vi "Actor Core.vi"(8 "error in":errorcluster, 11 "Main in":refnum<class "Main.lvclass">) -> (0 "error out":errorcluster, 3 "Actor out":refnum<class "Actor.lvclass">)   [LabVIEW 2025, in "Main.lvlib" / "Main.lvclass"]
doc: "<p>(<strong>Filename</strong>: <span class=\"dnl\">Actor Framework.lvlib:Actor.lvclass:Actor Core.vi</span>)</p>\n<p>Receives messages to the actor, reacts to them, and initiates any error handling that may shut the actor down.</p>\n<p>Descendant classes may override this VI to append parallel tasks for the actor to complete while it handles messages. Overrides use the <a href=\"nihelplauncher://docs/csh?context=lvcore_glang_udclass\">Call Parent Class Method</a> node.</p>"
uses:
  Main.lvclass
  C:/Program Files/National Instruments/LabVIEW 2025/vi.lib/ActorFramework/Actor/Actor.lvclass
  C:/Program Files/National Instruments/LabVIEW 2025/vi.lib/MGI/Panel Manager/Panel Actor/Panel Actor/Panel Actor.lvclass
  <vilib>/ActorFramework/Actor/Actor.lvclass
  File Worker/File Worker/File Worker.lvclass
  Main.lvclass/Main.ctl
  <vilib>/ActorFramework/Message Enqueuer/Message Enqueuer.lvclass/Message Enqueuer.ctl
  File Worker/File Worker Messages/Start Write Action Msg/Start Write Action Msg.lvclass/Start Write Action Msg.ctl
  File Worker/File Worker Messages/Start Read Action Msg/Start Read Action Msg.lvclass/Start Read Action Msg.ctl
  08b86284-690f-4d6a-a57b-caf26b63b25f.vi
  <vilib>/ActorFramework/Message Enqueuer/Enqueue.vi
  <vilib>/ActorFramework/Stop Msg/Stop Msg.lvclass
  C:/Program Files/National Instruments/LabVIEW 2025/vi.lib/ActorFramework/Message/Message.lvclass
  Main Messages/Reset Write Statistics Msg/Reset Write Statistics Msg.lvclass
  File Worker/File Worker Messages/Start Write Action Msg/Start Write Action Msg.lvclass
  Main Messages/Reset Read Statistics Msg/Reset Read Statistics Msg.lvclass
  File Worker/File Worker Messages/Start Read Action Msg/Start Read Action Msg.lvclass
  <vilib>/ActorFramework/Message Priority Queue/Priority Enqueue.vi
  <vilib>/Platform/browser.llb/Open URL in Default Browser (string).vi
  <vilib>/MGI/Panel Manager/Panel Actor/Panel Actor/Panel Actor.lvclass
panel:
  in  "Visit RADX":bool
  in  "Visit G2CPU":bool
  in  "Stop Action":bool
  in  "Read":bool
  in  "Write":bool
  in  "Block Size":u16(ring)
  in  "Threads":i32=4 min=1 step=1
  in  "File Size":u16(ring)
  in  "Available Disks":u16(ring)
  out "Write Average":dbl format="%#_2g GB/s"
  out "Write Min":dbl format="%#_2g GB/s"
  out "Write Max":dbl format="%#_2g GB/s"
  out "Write Plot":waveform(dbl)(graph)
  out "Read Average":dbl format="%#_2g GB/s"
  out "Read Min":dbl format="%#_2g GB/s"
  out "Read Max":dbl format="%#_2g GB/s"
  out "Read Plot":waveform(dbl)(graph)
  # "GPU acceleration in LabVIEW?"
  # "Sponsored by:"
  # "COTS, High Performance PXIe Data Storage, GPU and GbE"
  # "Copyright 2025 G2CPU, Ltd. \nAll Rights Reserved."
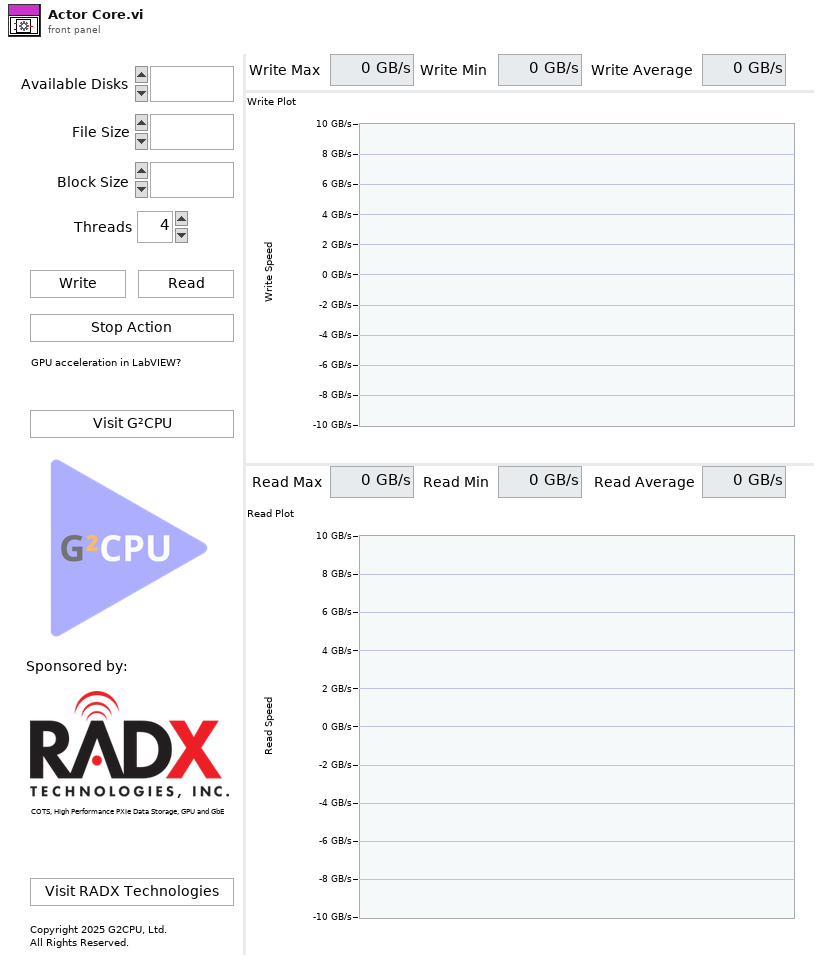
[diagram p1: front panel]
types:
  T1 = enum32{"Invalid", "Standard", "Closed", "Hidden", "Minimized", "Maximized"}
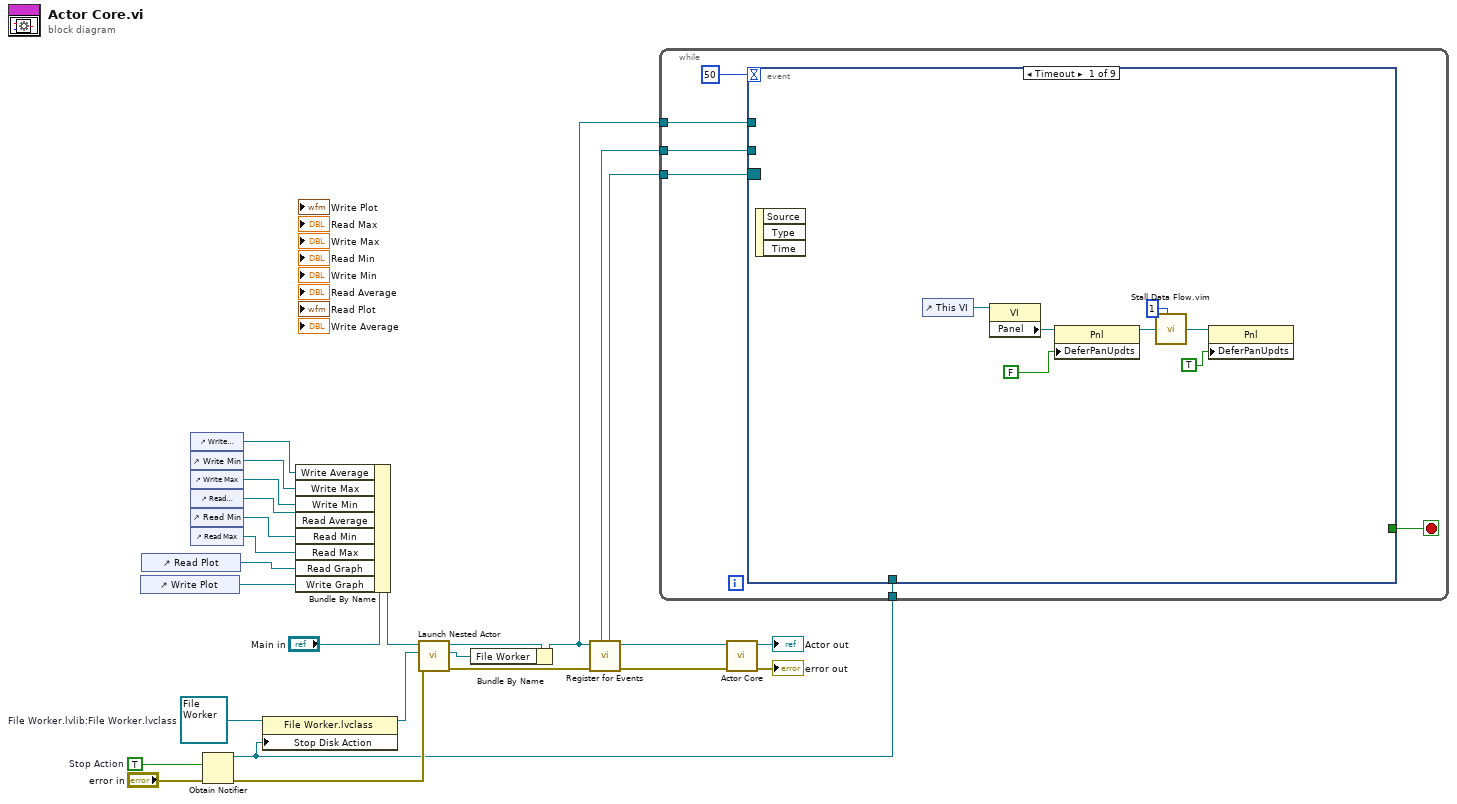
[diagram p0: block diagram]
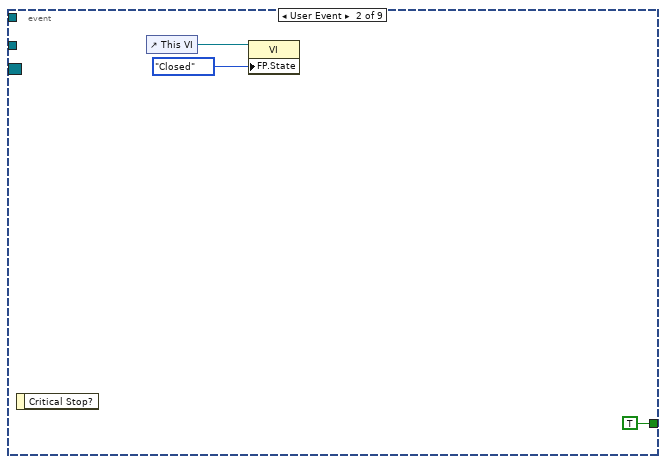
[diagram p2: hidden frame]
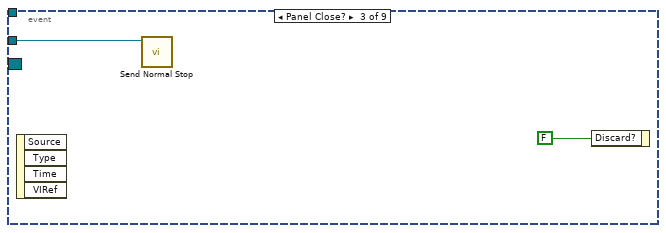
[diagram p3: hidden frame]
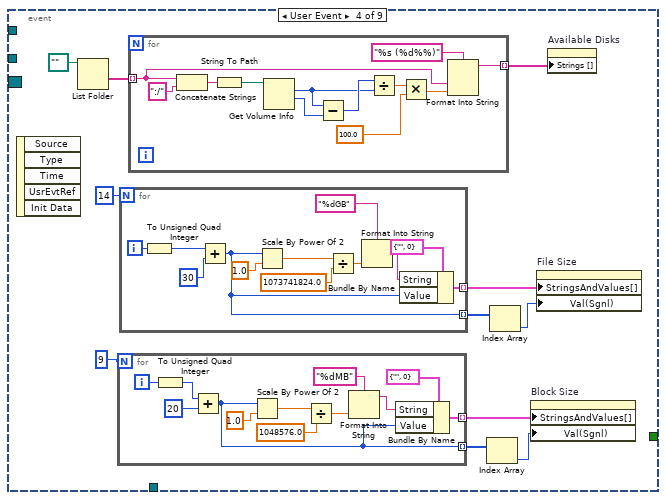
[diagram p4: hidden frame]
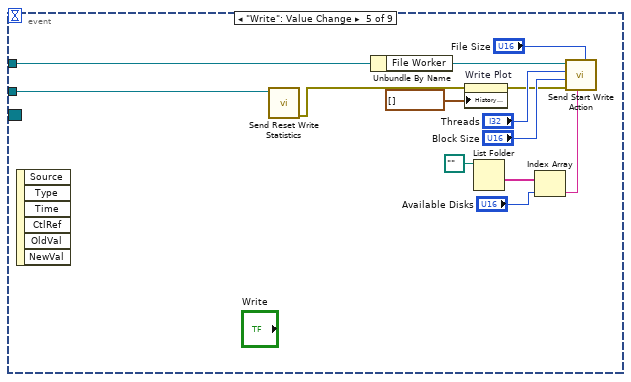
[diagram p5: hidden frame]
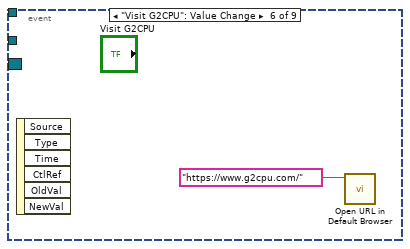
[diagram p6: hidden frame]
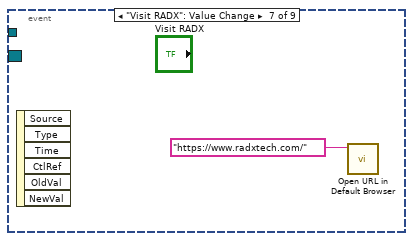
[diagram p7: hidden frame]
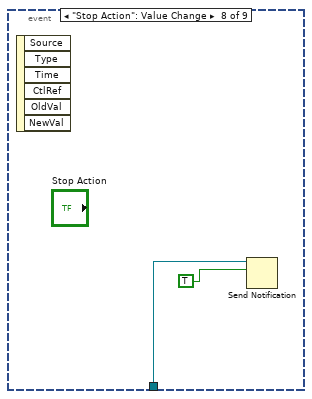
[diagram p8: hidden frame]
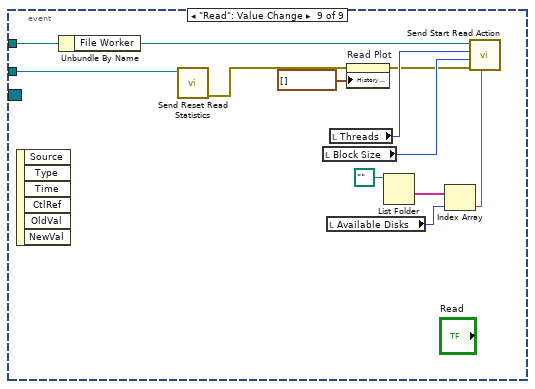
[diagram p9: hidden frame]
diagram:
  w11 = TRUE  # Stop Action
  w17 = refnum<class "File Worker.lvclass"> refnum  # File Worker.lvlib:File Worker.lvclass
  n1 = control-ref of="Write Plot"() -> (w13:refnum<vi>)
  n2 = control-ref of="Read Plot"() -> (w12:refnum<vi>)
  n3 = control-ref of="Write Average"() -> (w6:refnum<vi>)
  n4 = control-ref of="Write Min"() -> (w5:refnum<vi>)
  n5 = control-ref of="Write Max"() -> (w4:refnum<vi>)
  n6 = control-ref of="Read Average"() -> (w3:refnum<vi>)
  n7 = control-ref of="Read Min"() -> (w2:refnum<vi>)
  n8 = control-ref of="Read Max"() -> (w1:refnum<vi>)
  n9 = Obtain Notifier(notification data type=w11, error in (no error)="error in") -> (notifier out=w7:refnum<notifier>, error out=w9:errorcluster)  [unwired: 2 in, 1 out]
  n10 = property class="File Worker.lvclass"(reference=w17, "Stop Disk Action"=w7) -> (reference out=w8:refnum<class "File Worker.lvclass">)  [unwired: 1 in, 1 out]
  n11 = Bundle By Name(cluster="Main in", "Write Average"=w6, "Write Max"=w5, "Write Min"=w4, "Read Average"=w3, "Read Min"=w2, "Read Max"=w1, "Read Graph"=w12, "Write Graph"=w13) -> (w14:refnum<class "Main.lvclass">)
  n12 = call <vilib>:"Launch Nested Actor.vi"("error in (no error)"=w9, "Nested Actor"=w8, "Caller Actor in"=w14) -> ("error out"=w20:errorcluster, "Nested Actor's Enqueuer"=w16:refnum<class "Message Enqueuer.lvclass">, "Caller Actor out"=w18:refnum<class "Main.lvclass">)  [unwired: 6 in]
  n13 = Bundle By Name(cluster=w18, "File Worker"=w16) -> (w15:refnum<class "Main.lvclass">)
  n14 = call <vilib>:"Register for Events.vi"("Error In"=w20, "Panel Actor in"=w15) -> ("Error Out"=w23:errorcluster, "Panel Actor out"=w24:refnum<class "Main.lvclass">, "Pnl Actor"=w22:refnum<event-registration>, "Self Enqueuer"=w21:refnum<class "Message Enqueuer.lvclass">)  [unwired: 6 in]
  n15 = while {
    tunnel: w22 -> [w32]
    tunnel: w21 -> [w30]
    tunnel: w15 -> [w29]
    tunnel: w7 -> [w28]
    stop <- w31 stop-if-true
    n16 = event shown="[0] Timeout" {
      selector: w32 -> [_ _ _ _ _ _ _ _ _]
      dyn-events: _ -> [_ _ _ _ _ _ _ _ _]
      timeout: 50 -> [_ _ _ _ _ _ _ _ _]
      tunnel: [_ TRUE _ _ _ _ _ _ _] -> w31
      tunnel: w30 -> [_ _ w43 _ w93 _ _ _ w109]
      tunnel: w29 -> [_ _ _ _ w104 _ _ _ w120]
      tunnel: w28 -> [_ _ _ _ _ _ _ w108 _]
      event Timeout {
        n17 = event-data() -> ()  [unwired: 1 in, 3 out]
        n18 = control-ref of="This VI"() -> (w38:refnum<vi>)
        n19 = property class="VI"(reference=w38) -> ("Panel"=w39:refnum<vi>)  [unwired: 1 in, 2 out]
        n20 = property class="Pnl"(reference=w39, "DeferPanUpdts"=FALSE ("Defer Panel Updates")) -> (reference out=w36:refnum<vi>)  [unwired: 1 in, 1 out]
        n21 = call "Stall Data Flow.vim"("value in"=w36, "milliseconds to wait"=u32 1) -> ("value out"=w34:refnum<vi>)  [unwired: 1 out]
        n22 = property class="Pnl"(reference=w34, "DeferPanUpdts"=TRUE ("Defer Panel Updates")) -> ()  [unwired: 1 in, 2 out]
      }
      event User Event {
        n23 = event-data() -> ()  [unwired: 1 in, 1 out]
        n24 = control-ref of="This VI"() -> (w41:refnum<vi>)
        n25 = property class="VI"(reference=w41, "FP.State"=T1."Closed" ("Front Panel Window:State")) -> ()  [unwired: 1 in, 2 out]
      }
      event Panel Close? {
        n26 = event-data() -> ()  [unwired: 1 in, 4 out]
        n27 = call <vilib>:"Send Normal Stop.vi"("Message Enqueuer"=w43) -> ()  [unwired: 10 in, 1 out]
        n28 = event-data("Discard?"=FALSE) -> ()  [unwired: 1 in, 1 out]
      }
      event User Event {
        n29 = event-data() -> ()  [unwired: 1 in, 5 out]
        n30 = List Folder(path=path "") -> (folder names=w54:string[])  [unwired: 3 in, 3 out]
        n31 = for {
          N: 9 -> [_]
          tunnel: [w58] -> w47 mode=indexing
          tunnel: [w56] -> w45 mode=indexing
          i -> [w62]
          n32 = To Unsigned Quad Integer(1:w62) -> (0:w57:u64)
          n33 = Add(x=w57, y=u64 20) -> (x+y=w56:u64)
          n34 = Scale By Power Of 2(n=w56, x=1.0 ("y")) -> (x*2^n=w67:dbl)
          n35 = Divide(x=w67, y=1048576.0 ("x")) -> (x/y=w61:dbl)
          n36 = Format Into String(format string="%dMB", w61) -> (resulting string=w59:string)  [unwired: 2 in, 1 out]
          n37 = Bundle By Name(cluster=cluster{"String":string, "Value":u16} {"String"="", "Value"=0} ("element"), "String"=w59, "Value"=w56) -> (w58:cluster{"String":string, "Value":u16})
        }
        n38 = for {
          N: 14 -> [_]
          tunnel: [w72] -> w51 mode=indexing
          tunnel: [w69] -> w50 mode=indexing
          i -> [w78]
          n39 = To Unsigned Quad Integer(1:w78) -> (0:w68:u64)
          n40 = Add(x=w68, y=u64 30) -> (x+y=w69:u64)
          n41 = Scale By Power Of 2(n=w69, x=1.0 ("y")) -> (x*2^n=w73:dbl)
          n42 = Divide(x=w73, y=1073741824.0 ("x")) -> (x/y=w71:dbl)
          n43 = Format Into String(format string="%dGB", w71) -> (resulting string=w74:string)  [unwired: 2 in, 1 out]
          n44 = Bundle By Name(cluster=cluster{"String":string, "Value":u16} {"String"="", "Value"=0} ("element"), "String"=w74, "Value"=w69) -> (w72:cluster{"String":string, "Value":u16})
        }
        n45 = for {
          tunnel: w54 -> [w82] mode=indexing
          tunnel: [w80] -> w53 mode=indexing
          n46 = Concatenate Strings(w82, ":/" ("string")) -> (w90:string)
          n47 = String To Path(string=w90) -> (path=w91:path)
          n48 = Get Volume Info(11:w91) -> (1:w88:i64, 2:w86:i64)  [unwired: 1 in, 4 out]
          n49 = Subtract(x=w86, y=w88) -> (x-y=w87:i64)
          n50 = Divide(x=w87, y=w86) -> (x/y=w85:dbl)
          n51 = Multiply(x=w85, y=100.0) -> (x*y=w81:dbl)
          n52 = Format Into String(format string="%s (%d%%)", w82, w81) -> (resulting string=w80:string)  [unwired: 2 in, 1 out]
        }
        n53 = Index Array(array=w45) -> (element=w46:u64)  [unwired: 1 in]
        n54 = Index Array(array=w50) -> (element=w49:u64)  [unwired: 1 in]
        n55 = property on="Block Size" class="Ring (strict)"("StringsAndValues[]"=w47, "Val(Sgnl)"=w46) -> ()  [unwired: 2 in, 2 out]
        n56 = property on="File Size" class="Ring (strict)"("StringsAndValues[]"=w51, "Val(Sgnl)"=w49) -> ()  [unwired: 2 in, 2 out]
        n57 = property on="Available Disks" class="Ring (strict)"("Strings []"=w53) -> ()  [unwired: 2 in, 2 out]
      }
      event "Write": Value Change {
        n58 = event-data() -> ()  [unwired: 1 in, 6 out]
        n59 = call "Send Reset Write Statistics.vi"("Message Enqueuer"=w93) -> ("error out"=w92:errorcluster)  [unwired: 9 in, 1 out]
        n60 = Unbundle By Name(w104) -> ("File Worker"=w103:refnum<class "Message Enqueuer.lvclass">)
        n61 = property on="Write Plot" class="WFChart (strict)"(error in=w92, "History Data"=waveform(dbl)[] []) -> (error out=w95:errorcluster)  [unwired: 1 in, 1 out]
        n62 = List Folder(path=path "") -> (folder names=w96:string[])  [unwired: 3 in, 3 out]
        n63 = Index Array(array=w96, index="Available Disks") -> (element=w98:string)
        n64 = call "Send Start Write Action.vi"("File Size"="File Size", "Disk"=w98, "error in (no error)"=w95, "Block Size"="Block Size", "Thread"="Threads", "Message Enqueuer"=w103) -> ()  [unwired: 4 in, 2 out]
      }
      event "Visit G2CPU": Value Change {
        n65 = event-data() -> ()  [unwired: 1 in, 6 out]
        n66 = call-poly <vilib>:"Open URL in Default Browser.vi"("URL"="https://www.g2cpu.com/") -> ()  [unwired: 5 in, 2 out]
      }
      event "Visit RADX": Value Change {
        n67 = event-data() -> ()  [unwired: 1 in, 6 out]
        n68 = call-poly <vilib>:"Open URL in Default Browser.vi"("URL"="https://www.radxtech.com/") -> ()  [unwired: 5 in, 2 out]
      }
      event "Stop Action": Value Change {
        n69 = event-data() -> ()  [unwired: 1 in, 6 out]
        n70 = Send Notification(notification=TRUE, notifier=w108) -> ()  [unwired: 1 in, 2 out]
      }
      event "Read": Value Change {
        n71 = event-data() -> ()  [unwired: 1 in, 6 out]
        n72 = Unbundle By Name(w120) -> ("File Worker"=w116:refnum<class "Message Enqueuer.lvclass">)
        n73 = call "Send Reset Read Statistics.vi"("Message Enqueuer"=w109) -> ("error out"=w110:errorcluster)  [unwired: 9 in, 1 out]
        n74 = local read "Block Size"() -> (w114:u16)
        n75 = local read "Available Disks"() -> (w112:u16)
        n76 = local read "Threads"() -> (w115:i32)
        n77 = property on="Read Plot" class="WFChart (strict)"(error in=w110, "History Data"=waveform(dbl)[] []) -> (error out=w111:errorcluster)  [unwired: 1 in, 1 out]
        n78 = List Folder(path=path "") -> (folder names=w118:string[])  [unwired: 3 in, 3 out]
        n79 = Index Array(array=w118, index=w112) -> (element=w113:string)
        n80 = call "Send Start Read Action.vi"("Disk"=w113, "error in (no error)"=w111, "Block Size"=w114, "Thread"=w115, "Message Enqueuer"=w116) -> ()  [unwired: 5 in, 2 out]
      }
    }
  }
  n81 = call-parent "Actor Core.vi"("error in"=w23, "Panel Actor in"=w24) -> ("error out"=→"error out":errorcluster, "Actor out"=→"Actor out":refnum<class "Actor.lvclass">)  [unwired: 8 in]
